vi "GetTorqueWfmDataSetProps.vi"(6 "do not write to database":bool, 8 "error in (no error)":errorcluster, 10 "waveform":waveform(sgl), 11 "dataset props in":T1[](array[typedef])) -> (0 "error out":errorcluster, 3 "dataset props out":T1[](array[typedef]))   [LabVIEW 2017, in "McsaDataEventCreator.lvlib"]
uses:
  <vilib>/addons/InsightCM/Devices/Shared/Mcsa/McsaDataEventCreator/McsaDataEventCreator.lvlib
  <vilib>/addons/InsightCM/MessageBus/Base/controls/KeyValuePair.ctl
  <vilib>/addons/InsightCM/Devices/Shared/Common/DataEventCreator/DataEventCreator.lvlib
  <vilib>/addons/InsightCM/Utilities/PropertyHelpers/PropertyHelpers.lvlib
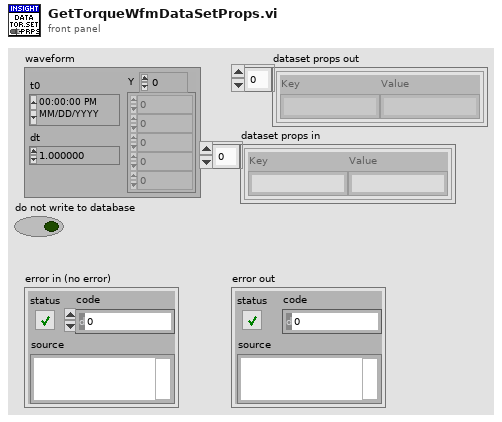
[diagram p1: front panel]
types:
  T1 = typedef "KeyValuePair.ctl" = cluster{"Key":string, "Value":string}
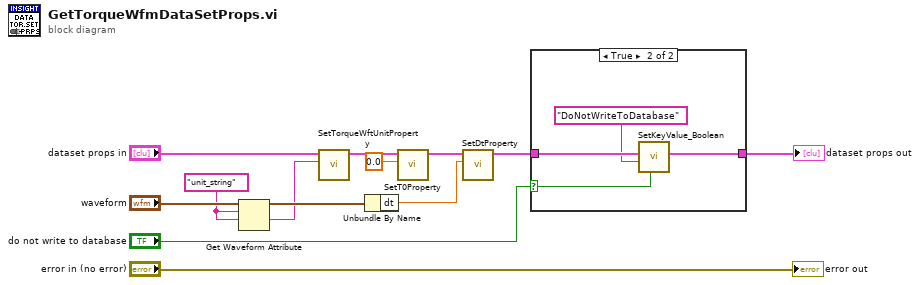
[diagram p0: block diagram]
diagram:
  w1 = "unit_string" ("name")
  n1 = Get Waveform Attribute(5:w1, 6:w1, 7:"waveform") -> (1:w2:string, 3:w5:waveform(sgl))  [unwired: 1 in, 2 out]
  n2 = call <vilib>:"SetTorqueWftUnitProperty.vi"("unit_string"=w2, "props in"="dataset props in") -> ("props out"=w3:T1[])  [unwired: 9 in]
  n3 = Unbundle By Name(w5) -> ("dt"=w13:dbl)
  n4 = call <vilib>:"SetT0Property.vi"("Toffset"=0.0 ("T0"), "props in"=w3) -> ("props out"=w9:T1[])  [unwired: 9 in]
  n5 = call <vilib>:"SetDtProperty.vi"("dt"=w13, "props in"=w9) -> ("props out"=w12:T1[])  [unwired: 9 in]
  n6 = case shown="True" "do not write to database" {
    selector: "do not write to database" -> [_ w15]
    tunnel: w12 -> [w14 w18]
    tunnel: [w14 w17] -> w11
    frame False {
    }
    frame True {
      n7 = call <vilib>:"SetKeyValue_Boolean.vi"("value"=w15, "key"="DoNotWriteToDatabase", "key value pairs"=w18) -> ("key value pairs out"=w17:T1[])  [unwired: 8 in]
    }
  }
  "dataset props out" <- w11
  "error out" <- "error in (no error)"
